vi "Check Path (word).vi"(2 "error in (no error)":errorcluster, 3 "path in":path) -> (0 "error out":errorcluster, 1 "path out":path)   [LabVIEW 2010, in "NI_ReportGenerationToolkit.lvlib"]
doc: "Checks the path to see if it actually exists on disk. If it does not the error cluster is set. If the path is a relative path, an absolute path is made from the relative path by appending it with the path to the directory in which the top most VI of this program exists."
uses:
  <vilib>/addons/_office/NI_ReportGenerationToolkit.lvlib
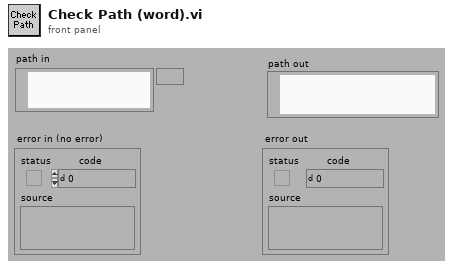
[diagram p1: front panel]
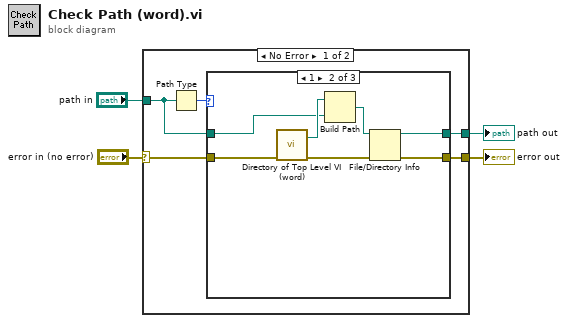
[diagram p0: block diagram]
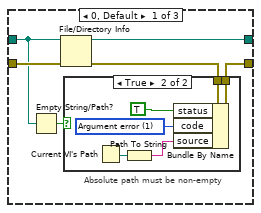
[diagram p2: hidden frame]
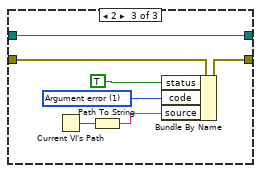
[diagram p4: hidden frame]
diagram:
  n1 = case shown="No Error" "error in (no error)" {
    selector: "error in (no error)" -> [w5 w38]
    tunnel: [w8 w38] -> w4
    tunnel: "path in" -> [w7 w37]
    tunnel: [w6 w37] -> w2
    frame No Error {
      n2 = Path Type(1:w7) -> (0:w9:i16)
      n3 = case shown="1" w9 {
        tunnel: w5 -> [w15 w29 w32]
        tunnel: [w12 w24 w31] -> w8
        tunnel: w7 -> [w11 w27 w30]
        tunnel: [w14 w23 w30] -> w6
        frame 0, Default {
          # "Absolute path must be non-empty"
          n4 = Empty String/Path?(string/path=w11) -> (empty?=w10:bool)
          n5 = File/Directory Info(path=w11, error in=w15) -> (path out=w14:path, error out=w13:errorcluster)  [unwired: 5 out]
          n6 = case shown="True" w10 {
            tunnel: w13 -> [w16 w18]
            tunnel: [w16 w17] -> w12
            frame False {
            }
            frame True {
              w20 = 1 items=["No error", "Argument error", "Memory is full", "Out of zone", "End of file", "File already open", "Generic file I/O error", "File not found", "File permission error", "Disk is full", "Duplicate path", "Too many files open", "System feature not enabled", "Resource file not found", "Cannot add resource", "Resource not found", "Image not found", "Image memory error", "Pen does not exist", "Config type invalid", "Config token not found", "Config parse error", "Config memory error", "Bad external code format", "Bad external code offset", "External code not present", "Null window", "Destroy window error", "Null menu", "Print aborted", "Bad print record", "Print driver error", "Windows error during printing", "Memory error during printing", "Print dialog error", "Generic print error", "Invalid device refnum", "Device not found", "Device parameter error", "Device unit error", "Cannot open device", "Device call aborted", "Generic error", "Cancelled by user", "Object ID too low", "Object ID too high", "Object not in heap", "Unknown heap", "Unknown object (invalid DefProc)", "Unknown object (DefProc not in table)", "Message out of range", "Invalid (null) method", "Unknown message", "Manager call not supported", "Bad address", "Network operation in progress", "Network operation timed out", "Connection is busy", "Network attribute not supported", "Network error", "Address in use", "System out of memory", "Connection aborted", "Connection refused", "Not connected", "Already connected", "Connection closed", "Initialization error (interapplication manager)", "Bad occurrence", "Wait on unbound occurrence handler", "Occurrence queue overflow", "Datalog type conflict", "Unused", "Unrecognized type (interapplication manager)", "Memory corrupt", "Failed to make temporary DLL", "Old CIN version", "Drag socket not found", "Failed to load drop-object", "Failed to register OLE object", "Failed to release OLE object", "Format specifier type mismatch", "Unknown format specifier", "Too few format specifiers", "Too many format specifiers", "Scan failed", "Newer CIN version", "Error converting to variant", "Runtime menu error", "Password tampered", "Variant attribute not found", "Incompatible variant data type", "Event data is not available", "Event Store is not present", "Occurrence is not found", "Event Queue is not created", "Event info is not available", "Refnum passed is NULL", "Error retrieving Class GUID", "Error retrieving CoClass GUID", "Error retrieving TypeLib GUID.", "Bad built application magic bytes.", "Specific driver is different from the specific driver associated with the Logical Name.", "There is no session opened to the class driver.", "Max Error", "MAX - Error with config objects", "MAX - Error loading configuration", "MAX - Group not supported"]
              n7 = Current VI's Path() -> (path=w21:path)
              n8 = Path To String(path=w21) -> (string=w22:string)
              n9 = Bundle By Name(cluster=w18, "status"=TRUE, "code"=w20, "source"=w22) -> (w17:errorcluster)
            }
          }
        }
        frame 1 {
          n10 = call <vilib>:"Directory of Top Level VI (word).vi"("error in (no error)"=w29) -> ("directory of top VI"=w28:path, "error out"=w25:errorcluster)
          n11 = Build Path(base path=w28, name or relative path=w27) -> (appended path=w26:path)
          n12 = File/Directory Info(path=w26, error in=w25) -> (path out=w23:path, error out=w24:errorcluster)  [unwired: 5 out]
        }
        frame 2 {
          w34 = 1 items=["No error", "Argument error", "Memory is full", "Out of zone", "End of file", "File already open", "Generic file I/O error", "File not found", "File permission error", "Disk is full", "Duplicate path", "Too many files open", "System feature not enabled", "Resource file not found", "Cannot add resource", "Resource not found", "Image not found", "Image memory error", "Pen does not exist", "Config type invalid", "Config token not found", "Config parse error", "Config memory error", "Bad external code format", "Bad external code offset", "External code not present", "Null window", "Destroy window error", "Null menu", "Print aborted", "Bad print record", "Print driver error", "Windows error during printing", "Memory error during printing", "Print dialog error", "Generic print error", "Invalid device refnum", "Device not found", "Device parameter error", "Device unit error", "Cannot open device", "Device call aborted", "Generic error", "Cancelled by user", "Object ID too low", "Object ID too high", "Object not in heap", "Unknown heap", "Unknown object (invalid DefProc)", "Unknown object (DefProc not in table)", "Message out of range", "Invalid (null) method", "Unknown message", "Manager call not supported", "Bad address", "Network operation in progress", "Network operation timed out", "Connection is busy", "Network attribute not supported", "Network error", "Address in use", "System out of memory", "Connection aborted", "Connection refused", "Not connected", "Already connected", "Connection closed", "Initialization error (interapplication manager)", "Bad occurrence", "Wait on unbound occurrence handler", "Occurrence queue overflow", "Datalog type conflict", "Unused", "Unrecognized type (interapplication manager)", "Memory corrupt", "Failed to make temporary DLL", "Old CIN version", "Drag socket not found", "Failed to load drop-object", "Failed to register OLE object", "Failed to release OLE object", "Format specifier type mismatch", "Unknown format specifier", "Too few format specifiers", "Too many format specifiers", "Scan failed", "Newer CIN version", "Error converting to variant", "Runtime menu error", "Password tampered", "Variant attribute not found", "Incompatible variant data type", "Event data is not available", "Event Store is not present", "Occurrence is not found", "Event Queue is not created", "Event info is not available", "Refnum passed is NULL", "Error retrieving Class GUID", "Error retrieving CoClass GUID", "Error retrieving TypeLib GUID.", "Bad built application magic bytes.", "Specific driver is different from the specific driver associated with the Logical Name.", "There is no session opened to the class driver.", "Max Error", "MAX - Error with config objects", "MAX - Error loading configuration", "MAX - Group not supported"]
          n13 = Current VI's Path() -> (path=w35:path)
          n14 = Path To String(path=w35) -> (string=w36:string)
          n15 = Bundle By Name(cluster=w32, "status"=TRUE, "code"=w34, "source"=w36) -> (w31:errorcluster)
        }
      }
    }
    frame Error {
    }
  }
  "error out" <- w4
  "path out" <- w2
